vi "DI A Faults.vi"(9 "FIFO Indexes":T2[](array[typedef]), 10 "A DI Faults":T1[](array[typedef]), 11 "Device Outputs in":dbl[](array[numeric])) -> (3 "Device Outputs out":dbl[](array[numeric]))   [LabVIEW 2016, in "DCM Engine.lvlib"]
uses:
  DCM Engine.lvlib
  Shared/Types/DI Faults Indexes.ctl
  <vilib>/Powertrain Controls/Device Drivers/DCM/Rev0/FPGA/DI - Faults.ctl
  DCM Shared.lvlib
  <vilib>/Powertrain Controls/Device Drivers/DCM/Rev0/FPGA/DCM - FPGA.lvlib
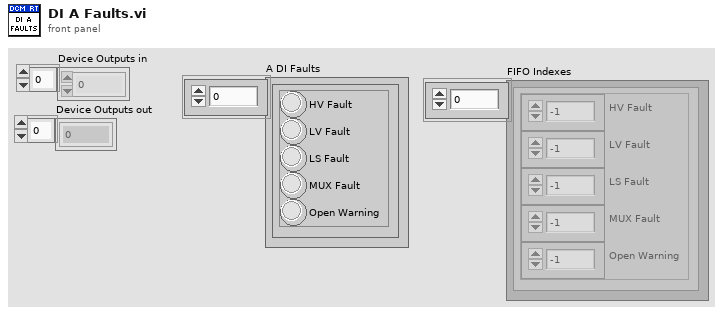
[diagram p1: front panel]
types:
  T1 = typedef "DCM - FPGA.lvlib/DI - Faults.ctl" = cluster{"HV Fault":bool, "LV Fault":bool, "LS Fault":bool, "MUX Fault":bool, "Open Warning":bool}
  T2 = typedef "DCM Shared.lvlib/DI Faults Indexes.ctl" = cluster{"HV Fault":i32, "LV Fault":i32, "LS Fault":i32, "MUX Fault":i32, "Open Warning":i32}
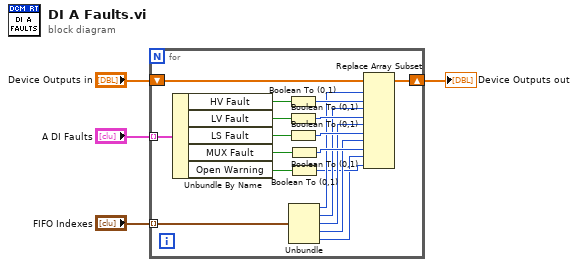
[diagram p0: block diagram]
diagram:
  n1 = for {
    tunnel: "A DI Faults" -> [w21] mode=indexing
    tunnel: "FIFO Indexes" -> [w12] mode=indexing
    shift-right: [w22] -> w1
    shift-left: "Device Outputs in" -> [w23]
    n2 = Unbundle By Name(w21) -> ("HV Fault"=w17:bool, "LV Fault"=w20:bool, "LS Fault"=w19:bool, "MUX Fault"=w18:bool, "Open Warning"=w7:bool)
    n3 = Boolean To (0,1)(Boolean=w17) -> (0, 1=w16:i16)
    n4 = Boolean To (0,1)(Boolean=w20) -> (0, 1=w15:i16)
    n5 = Boolean To (0,1)(Boolean=w19) -> (0, 1=w14:i16)
    n6 = Boolean To (0,1)(Boolean=w18) -> (0, 1=w13:i16)
    n7 = Boolean To (0,1)(Boolean=w7) -> (0, 1=w6:i16)
    n8 = Unbundle(w12) -> ("HV Fault"=w11:i32, "LV Fault"=w10:i32, "LS Fault"=w9:i32, "MUX Fault"=w8:i32, "Open Warning"=w5:i32)
    n9 = Replace Array Subset(array=w23, new element #1=w16, index #1=w11, new element #2=w15, index #2=w10, new element #3=w14, index #3=w9, new element #4=w13, index #4=w8, new element #5=w6, index #5=w5) -> (w22:dbl[])
  }
  "Device Outputs out" <- w1
